vi "GetAEStats.vi"(8 "Error In":errorcluster, 10 "SRs Out":T2[](array[typedef]), 11 "AE Name":string) -> (0 "Error Out":errorcluster, 1 "Survey Data Out  (Table)":string[][](array[string]), 2 "Survey Data Out (Raw)":T1, 3 "AE SRs Out":T2[](array[typedef]))   [LabVIEW 2017, in "DS_Lib.lvlib" / "SRReportParser.lvlib"]
uses:
  SRReportParser.lvlib
  TypeDefs/InWorkSR_Data.ctl
  TypeDefs/PR_Stats.ctl
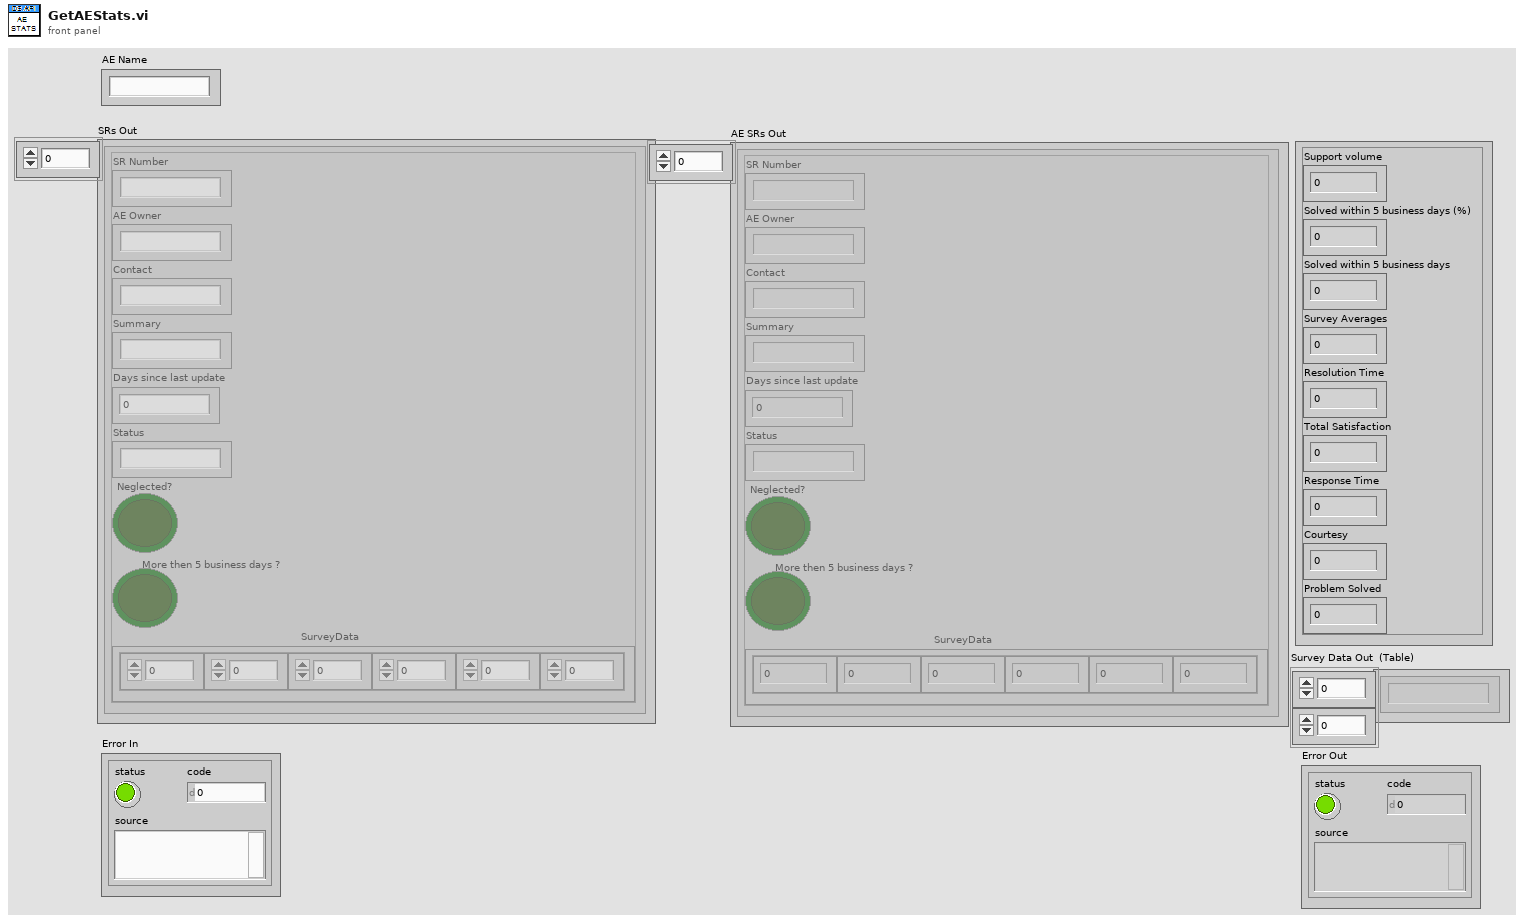
[diagram p1: front panel]
types:
  T1 = typedef "DS_Lib.lvlib/SRReportParser.lvlib/PR_Stats.ctl" = cluster{"Support volume":dbl, "Solved within 5 business days (%)":dbl, "Solved within 5 business days":dbl, "Survey Averages":dbl, "Resolution Time":dbl, "Total Satisfaction":dbl, "Response Time":dbl, "Courtesy":dbl, "Problem Solved":dbl}
  T2 = typedef "DS_Lib.lvlib/SRReportParser.lvlib/InWorkSR_Data.ctl" = cluster{"SR Number":string, "AE Owner":string, "Contact":string, "Summary":string, "Days since last update":dbl, "Status":string, "Neglected?":bool, "More then 5 business days ?":bool, "SurveyData":cluster{"Resolution Time":dbl, "Total Satisfaction":dbl, "Response Time":dbl, "Courtesy":dbl, "Problem Solved":dbl, "Level of effort":dbl}}
  T3 = cluster{"Resolution Time":dbl, "Total Satisfaction":dbl, "Response Time":dbl, "Courtesy":dbl, "Problem Solved":dbl, "Level of effort":dbl}
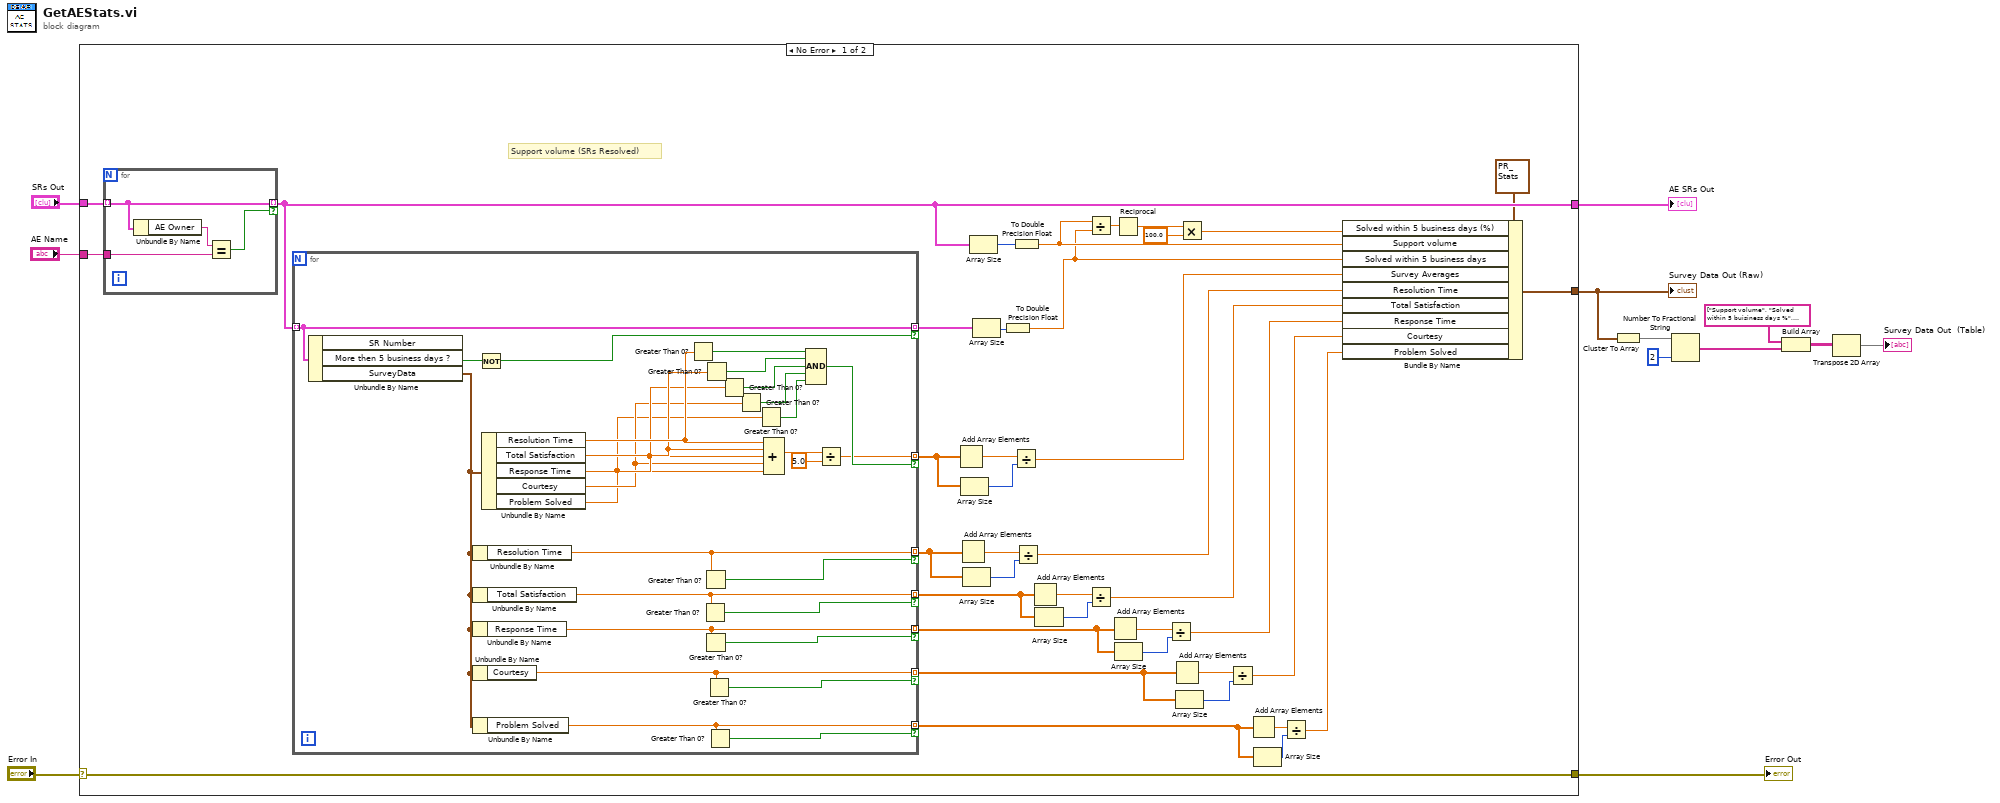
[diagram p0: block diagram]
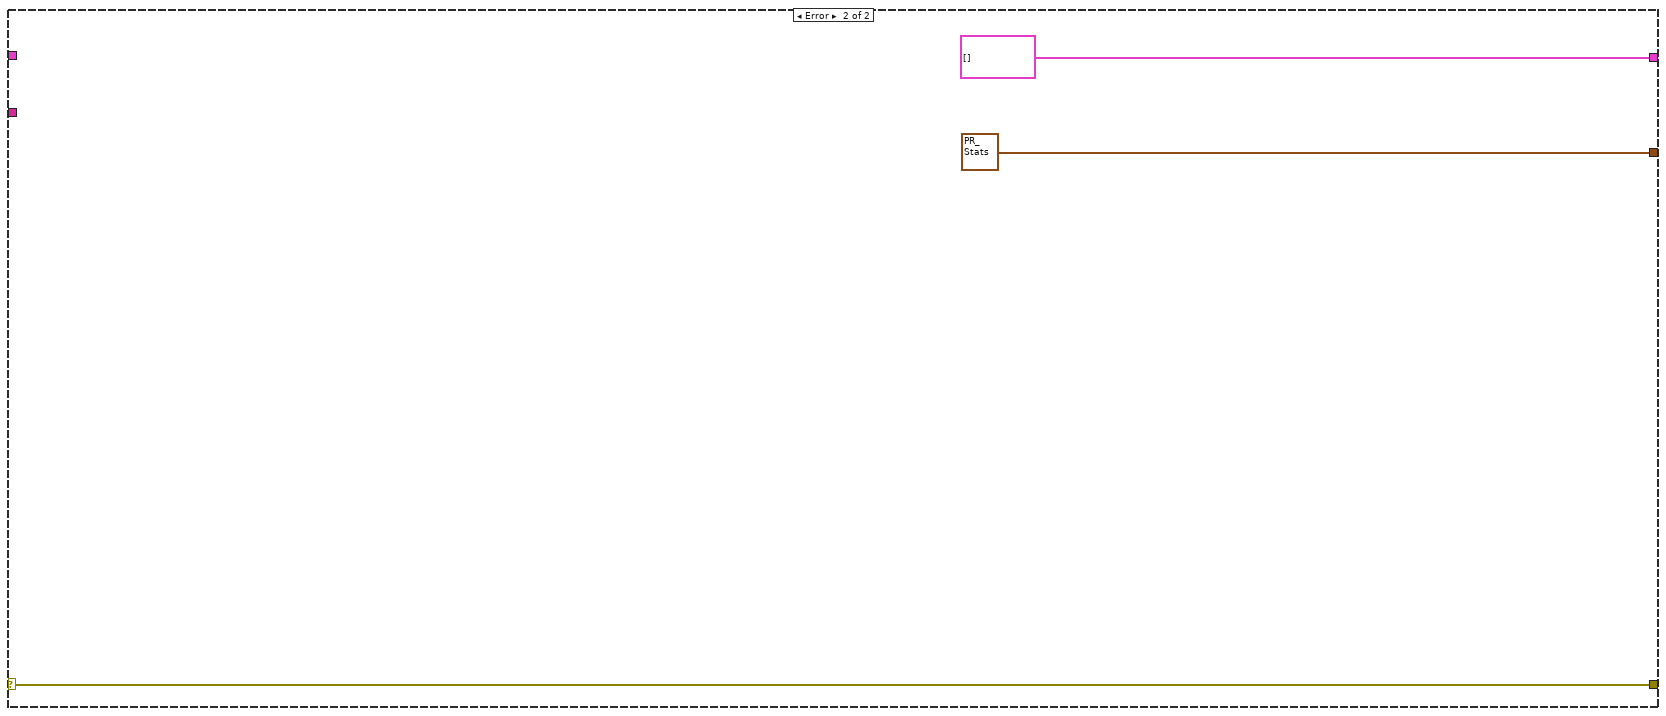
[diagram p2: hidden frame]
diagram:
  n1 = case shown="No Error" "Error In" {
    selector: "Error In" -> [w49 w86]
    tunnel: [w49 w86] -> w11
    tunnel: "SRs Out" -> [w51 _]
    tunnel: "AE Name" -> [w50 _]
    tunnel: [w48 T2[] []] -> w8
    tunnel: [w29 T1 {"Support volume"=0.0, "Solved within 5 business days (%)"=0.0, "Solved within 5 business days"=0.0, "Survey Averages"=0.0, "Resolution Time"=0.0, "Total Satisfaction"=0.0, "Response Time"=0.0, "Courtesy"=0.0, "Problem Solved"=0.0} ("Survey Data Out")] -> w7
    frame No Error {
      # "Support volume (SRs Resolved)"
      n2 = for {
        tunnel: w51 -> [w81] mode=indexing
        tunnel: w50 -> [w83]
        tunnel: [w81] -> w48 mode=indexing if=w80
        n3 = Unbundle By Name(w81) -> ("AE Owner"=w82:string)
        n4 = Equal?(x=w82, y=w83) -> (x = y?=w80:bool)
      }
      n5 = for {
        tunnel: w48 -> [w79] mode=indexing
        tunnel: [w79] -> w30 mode=indexing if=w77
        tunnel: [w52] -> w45 mode=indexing if=w66
        tunnel: [w65] -> w42 mode=indexing if=w64
        tunnel: [w63] -> w35 mode=indexing if=w62
        tunnel: [w61] -> w34 mode=indexing if=w60
        tunnel: [w58] -> w28 mode=indexing if=w57
        tunnel: [w55] -> w31 mode=indexing if=w56
        n6 = Unbundle By Name(w79) -> ("More then 5 business days ?"=w78:bool, "SurveyData"=w59:T3)  [unwired: 1 out]
        n7 = Unbundle By Name(w59) -> ("Resolution Time"=w65:dbl)
        n8 = Unbundle By Name(w59) -> ("Total Satisfaction"=w63:dbl)
        n9 = Unbundle By Name(w59) -> ("Response Time"=w61:dbl)
        n10 = Unbundle By Name(w59) -> ("Courtesy"=w58:dbl)
        n11 = Unbundle By Name(w59) -> ("Problem Solved"=w55:dbl)
        n12 = Not(x=w78) -> (.not. x?=w77:bool)
        n13 = Unbundle By Name(w59) -> ("Resolution Time"=w71:dbl, "Total Satisfaction"=w70:dbl, "Response Time"=w69:dbl, "Courtesy"=w68:dbl, "Problem Solved"=w67:dbl)
        n14 = Greater Than 0?(x=w71) -> (x > 0?=w76:bool)
        n15 = Greater Than 0?(x=w63) -> (x > 0?=w62:bool)
        n16 = Greater Than 0?(x=w65) -> (x > 0?=w64:bool)
        n17 = Greater Than 0?(x=w61) -> (x > 0?=w60:bool)
        n18 = Greater Than 0?(x=w70) -> (x > 0?=w75:bool)
        n19 = Greater Than 0?(x=w58) -> (x > 0?=w57:bool)
        n20 = Greater Than 0?(x=w55) -> (x > 0?=w56:bool)
        n21 = Greater Than 0?(x=w69) -> (x > 0?=w74:bool)
        n22 = Greater Than 0?(x=w68) -> (x > 0?=w73:bool)
        n23 = Greater Than 0?(x=w67) -> (x > 0?=w72:bool)
        n24 = Compound Arithmetic op=ADD(w71, w70, w69, w68, w67) -> (w54:dbl)
        n25 = Compound Arithmetic op=AND(w76, w75, w74, w73, w72) -> (w66:bool)
        n26 = Divide(x=w54, y=5.0) -> (x/y=w52:dbl)
      }
      n27 = Add Array Elements(numeric array=w45) -> (sum=w47:dbl)
      n28 = Add Array Elements(numeric array=w42) -> (sum=w43:dbl)
      n29 = Array Size(array=w45) -> (size(s)=w46:i32)
      n30 = Array Size(array=w42) -> (size(s)=w44:i32)
      n31 = Array Size(array=w48) -> (size(s)=w16:i32)
      n32 = Array Size(array=w30) -> (size(s)=w15:i32)
      n33 = To Double Precision Float(number=w15) -> (double precision float=w13:dbl)
      n34 = Divide(x=w47, y=w46) -> (x/y=w27:dbl)
      n35 = To Double Precision Float(number=w16) -> (double precision float=w14:dbl)
      n36 = Divide(x=w43, y=w44) -> (x/y=w26:dbl)
      n37 = Add Array Elements(numeric array=w35) -> (sum=w41:dbl)
      n38 = Array Size(array=w35) -> (size(s)=w40:i32)
      n39 = Divide(x=w14, y=w13) -> (x/y=w21:dbl)
      n40 = Divide(x=w41, y=w40) -> (x/y=w25:dbl)
      n41 = Add Array Elements(numeric array=w34) -> (sum=w38:dbl)
      n42 = Reciprocal(x=w21) -> (1/x=w20:dbl)
      n43 = Array Size(array=w34) -> (size(s)=w39:i32)
      n44 = Divide(x=w38, y=w39) -> (x/y=w24:dbl)
      n45 = Add Array Elements(numeric array=w28) -> (sum=w32:dbl)
      n46 = Array Size(array=w28) -> (size(s)=w33:i32)
      n47 = Multiply(x=w20, y=100.0) -> (x*y=w18:dbl)
      n48 = Divide(x=w32, y=w33) -> (x/y=w23:dbl)
      n49 = Add Array Elements(numeric array=w31) -> (sum=w37:dbl)
      n50 = Array Size(array=w31) -> (size(s)=w36:i32)
      n51 = Divide(x=w37, y=w36) -> (x/y=w22:dbl)
      n52 = Bundle By Name(cluster=T1 {"Support volume"=0.0, "Solved within 5 business days (%)"=0.0, "Solved within 5 business days"=0.0, "Survey Averages"=0.0, "Resolution Time"=0.0, "Total Satisfaction"=0.0, "Response Time"=0.0, "Courtesy"=0.0, "Problem Solved"=0.0} ("Survey Data Out"), "Solved within 5 business days (%)"=w18, "Support volume"=w14, "Solved within 5 business days"=w13, "Survey Averages"=w27, "Resolution Time"=w26, "Total Satisfaction"=w25, "Response Time"=w24, "Courtesy"=w23, "Problem Solved"=w22) -> (w29:T1)
    }
    frame Error {
    }
  }
  "Error Out" <- w11
  "AE SRs Out" <- w8
  "Survey Data Out (Raw)" <- w7
  n53 = Cluster To Array(cluster=w7) -> (array=w6:dbl[])
  n54 = Number To Fractional String(number=w6, precision (6)=i16 2) -> (F-format string=w3:string[])  [unwired: 2 in]
  n55 = Build Array(string[] ["Support volume", "Solved within 5 buisiness days %", "Solved within 5 buisiness days #", "Survey Averages", "Resolution Time", "Total Satisfactin", "Response Time", "Courtesy", "Problem Solved"] ("AE Statistics"), w3) -> (w2:string[][])
  n56 = Transpose 2D Array(2D array=w2) -> (transposed array=→"Survey Data Out  (Table)":string[][])
